vi "Actor Core.vi"(8 "error in":errorcluster, 11 "IEventHandler in":refnum<class "IEventHandler.lvclass">) -> (0 "error out":errorcluster, 3 "Actor out":refnum<class "Actor.lvclass">)   [LabVIEW 2020, in "MVA Framework.lvlib" / "ActorEvents.lvlib" / "IEventHandler.lvclass"]
doc: "(<B>Filename</B>: Actor Framework.lvlib:Actor.lvclass:Actor Core.vi)\n\nReceives messages to the actor, reacts to them, and initiates any error handling that may shut the actor down.\n\nDescendant classes may override this VI to append parallel tasks for the actor to complete while it handles messages. Overrides use the Call Parent Method node."
uses:
  IEventHandler.lvclass
  <vilib>/ActorFramework/Actor/Actor.lvclass
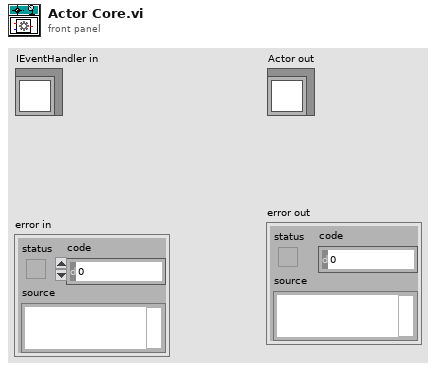
[diagram p1: front panel]
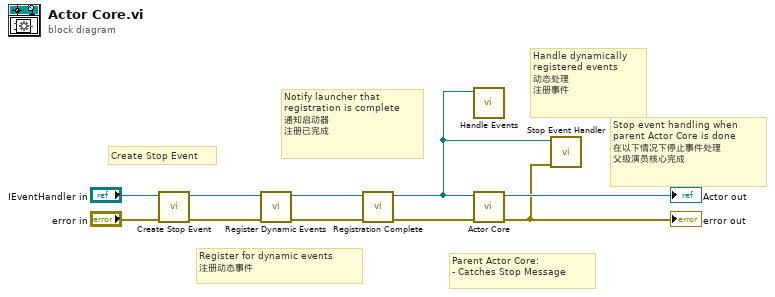
[diagram p0: block diagram]
diagram:
  # "Register for dynamic events\n注册动态事件"
  # "Notify launcher that\nregistration is complete\n通知启动器\n注册已完成"
  # "Handle dynamically\nregistered events\n动态处理\n注册事件"
  # "Stop event handling when\nparent Actor Core is done\n在以下情况下停止事件处理\n父级演员核心完成"
  # "Create Stop Event"
  # "Parent Actor Core:\n- Catches Stop Message"
  n1 = call "Create Stop Event.vi"("error in (no error)"="error in", "EventHandler"="IEventHandler in") -> ("error out"=w2:errorcluster, "EventHandler"=w7:refnum<class "IEventHandler.lvclass">)  [unwired: 8 in]
  n2 = call-dynamic "Register Dynamic Events.vi"("error in (no error)"=w2, "IEventHandler In"=w7) -> ("error out"=w1:errorcluster, "IEventHandler Out"=w3:refnum<class "IEventHandler.lvclass">)  [unwired: 8 in]
  n3 = call "Registration Complete.vi"("error in (no error)"=w1, "EventHandler"=w3) -> ("error out"=w4:errorcluster, "EventHandler"=w5:refnum<class "IEventHandler.lvclass">)  [unwired: 8 in]
  n4 = call-dynamic "Handle Events.vi"("EventHandler"=w5) -> ()  [unwired: 11 in]
  n5 = call-parent "Actor Core.vi"("error in"=w4, "Actor in"=w5) -> ("error out"=w6:errorcluster, "Actor out"=→"Actor out":refnum<class "Actor.lvclass">)  [unwired: 8 in]
  "error out" <- w6
  n6 = call "Stop Event Handler.vi"("error in (no error)"=w6, "EventHandler"=w5) -> ()  [unwired: 10 in]
